vi "refMgr_Example3.vi"() -> ()   [LabVIEW 2017]
uses:
  RefManager/Typedef/RefMgr-Logic-State.ctl
  RefManager/Typedef/RefMgr-StateChangeType.ctl
  RefManager/TagDB RefManager.lvlib
  <userlib>/_NEVSTOP/TagDB/TagDB.lvlib
  UIStateExpression/TagDB UIStateExpression.lvlib
panel:
  in  "aaa":string="aaaa"
  in  "toggle":bool
  in  "stop":bool
  in  "Boolean 0":bool
  in  "StateValue":i32
  in  "Boolean 5":bool
  in  "Boolean 4":bool
  in  "Boolean 3":bool
  in  "Boolean 2":bool
  in  "Boolean 1":bool
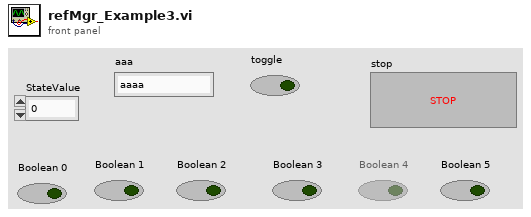
[diagram p1: front panel]
types:
  T1 = typedef "TagDB RefManager.lvlib/RefMgr-Logic-State.ctl" = cluster{"StateName":string, "StateValue":i32, "Type":T2, "Calcs":cluster{"Tag":string, "Exp":string}[]}
  T2 = typedef "TagDB RefManager.lvlib/RefMgr-StateChangeType.ctl" = enum16{"0 - 进入", "1 - 等于", "2 - 退出"}
  T3 = typedef "TagDB.lvlib/TagDB.ctl" = refnum<k1>
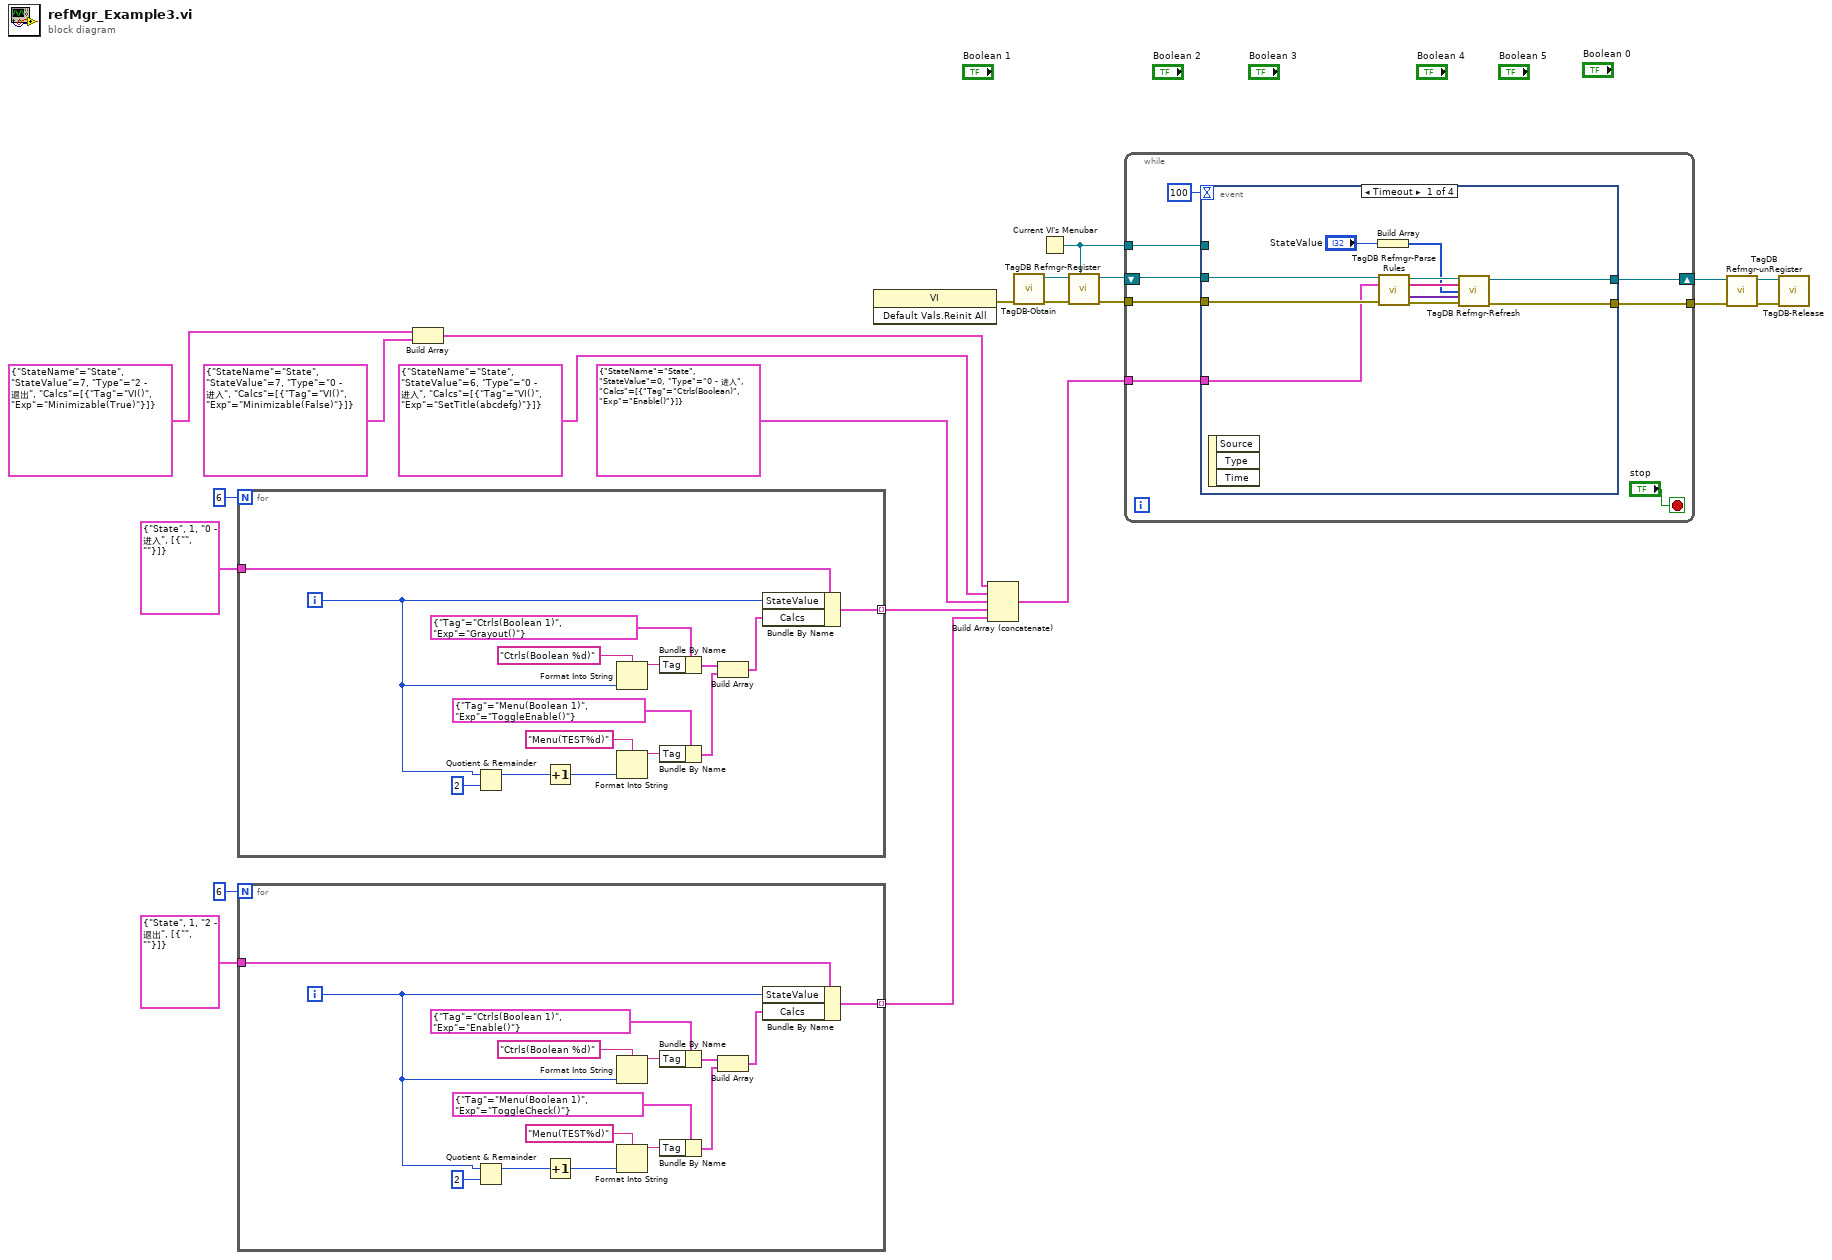
[diagram p0: block diagram]
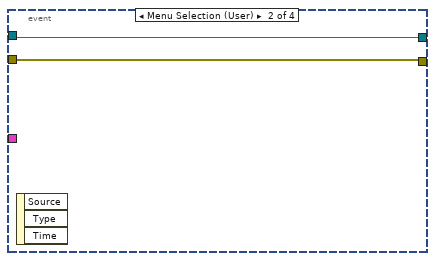
[diagram p2: hidden frame]
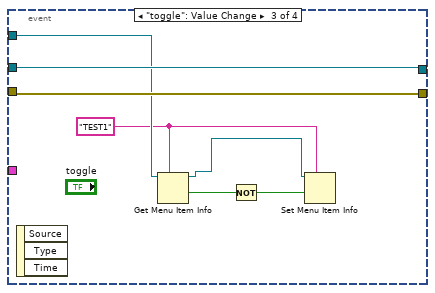
[diagram p3: hidden frame]
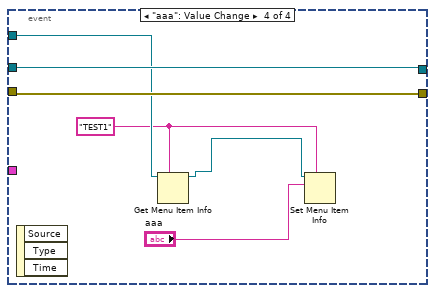
[diagram p4: hidden frame]
diagram:
  n1 = for {
    N: 6 -> [_]
    tunnel: T1 {"StateName"="State", "StateValue"=1, "Type"=enum."0 - 进入", "Calcs"=[{"Tag"="", "Exp"=""}]} ("Cluster") -> [w37]
    tunnel: [w31] -> w16 mode=indexing
    i -> [w27]
    n2 = Quotient & Remainder(x=w27, y=2) -> (x-y*floor(x/y)=w25:i32)  [unwired: 1 out]
    n3 = Increment(x=w25) -> (x+1=w23:i32)
    n4 = Format Into String(format string="Ctrls(Boolean %d)" ("Tag"), w27) -> (resulting string=w34:string)  [unwired: 2 in, 1 out]
    n5 = Format Into String(format string="Menu(TEST%d)" ("Tag"), w23) -> (resulting string=w30:string)  [unwired: 2 in, 1 out]
    n6 = Bundle By Name(cluster=cluster{"Tag":string, "Exp":string} {"Tag"="Ctrls(Boolean 1)", "Exp"="Grayout()"} ("Cluster"), "Tag"=w34) -> (w33:cluster{"Tag":string, "Exp":string})
    n7 = Bundle By Name(cluster=cluster{"Tag":string, "Exp":string} {"Tag"="Menu(Boolean 1)", "Exp"="ToggleEnable()"} ("Cluster"), "Tag"=w30) -> (w24:cluster{"Tag":string, "Exp":string})
    n8 = Build Array(w33, w24) -> (w32:cluster{"Tag":string, "Exp":string}[])
    n9 = Bundle By Name(cluster=w37, "StateValue"=w27, "Calcs"=w32) -> (w31:T1)
  }
  n10 = for {
    N: 6 -> [_]
    tunnel: T1 {"StateName"="State", "StateValue"=1, "Type"=enum."2 - 退出", "Calcs"=[{"Tag"="", "Exp"=""}]} ("Cluster") -> [w52]
    tunnel: [w46] -> w5 mode=indexing
    i -> [w42]
    n11 = Quotient & Remainder(x=w42, y=2) -> (x-y*floor(x/y)=w40:i32)  [unwired: 1 out]
    n12 = Increment(x=w40) -> (x+1=w38:i32)
    n13 = Format Into String(format string="Ctrls(Boolean %d)" ("Tag"), w42) -> (resulting string=w49:string)  [unwired: 2 in, 1 out]
    n14 = Format Into String(format string="Menu(TEST%d)" ("Tag"), w38) -> (resulting string=w45:string)  [unwired: 2 in, 1 out]
    n15 = Bundle By Name(cluster=cluster{"Tag":string, "Exp":string} {"Tag"="Ctrls(Boolean 1)", "Exp"="Enable()"} ("Cluster"), "Tag"=w49) -> (w48:cluster{"Tag":string, "Exp":string})
    n16 = Bundle By Name(cluster=cluster{"Tag":string, "Exp":string} {"Tag"="Menu(Boolean 1)", "Exp"="ToggleCheck()"} ("Cluster"), "Tag"=w45) -> (w39:cluster{"Tag":string, "Exp":string})
    n17 = Build Array(w48, w39) -> (w47:cluster{"Tag":string, "Exp":string}[])
    n18 = Bundle By Name(cluster=w52, "StateValue"=w42, "Calcs"=w47) -> (w46:T1)
  }
  n19 = Build Array(T1 {"StateName"="State", "StateValue"=7, "Type"=enum."2 - 退出", "Calcs"=[{"Tag"="VI()", "Exp"="Minimizable(True)"}]} ("Cluster"), T1 {"StateName"="State", "StateValue"=7, "Type"=enum."0 - 进入", "Calcs"=[{"Tag"="VI()", "Exp"="Minimizable(False)"}]} ("Cluster")) -> (w2:T1[])
  n20 = invoke class="VI" method="Default Vals.Reinit All"() -> (error out=w9:errorcluster)  [unwired: 3 in, 2 out]
  n21 = Build Array (concatenate)(w2, T1 {"StateName"="State", "StateValue"=6, "Type"=enum."0 - 进入", "Calcs"=[{"Tag"="VI()", "Exp"="SetTitle(abcdefg)"}]} ("Cluster"), T1 {"StateName"="State", "StateValue"=0, "Type"=enum."0 - 进入", "Calcs"=[{"Tag"="Ctrls(Boolean)", "Exp"="Enable()"}]} ("Cluster"), w16, w5) -> (w15:T1[])
  n22 = call <userlib>:"TagDB-Obtain.vi"("error in (no error)"=w9) -> ("error out"=w21:errorcluster, "TagDB"=w22:T3)  [unwired: 4 in, 1 out]
  n23 = Current VI's Menubar() -> (w8:refnum<k9>)
  n24 = call "TagDB Refmgr-Register.vi"("menu reference"=w8, "error in (no error)"=w21, "TagDB in"=w22) -> ("error out"=w19:errorcluster, "TagDB out"=w20:T3)  [unwired: 6 in, 1 out]
  n25 = while {
    tunnel: w19 -> [w59]
    tunnel: w15 -> [w58]
    tunnel: [w55] -> w12
    shift-right: [w56] -> w13
    shift-left: w20 -> [w60]
    tunnel: w8 -> [w53]
    stop <- "stop" stop-if-true
    n26 = event shown="[0] Timeout" {
      selector: _ -> [_ _ _ _]
      dyn-events: _ -> [_ _ _ _]
      timeout: 100 -> [_ _ _ _]
      tunnel: w60 -> [w71 w73 w80 w86]
      tunnel: w59 -> [w70 w72 w79 w85]
      tunnel: w58 -> [w69 _ _ _]
      tunnel: [w62 w73 w80 w86] -> w56
      tunnel: [w61 w72 w79 w85] -> w55
      tunnel: w53 -> [_ _ w77 w83]
      event Timeout {
        n27 = event-data() -> ()  [unwired: 1 in, 3 out]
        n28 = Build Array("StateValue") -> (w63:i32[])
        n29 = call "TagDB Refmgr-Parse Rules.vi"("DB Ref"=w71, "Rules"=w69, "error in (no error)"=w70) -> ("DB Ref (dup)"=w68:T3, "StateNames"=w66:string[], "RulesMap"=w65:variant[], "error out"=w67:errorcluster)  [unwired: 9 in]
        n30 = call "TagDB Refmgr-Refresh.vi"("DB Ref"=w68, "StateName"=w66, "State"=w63, "RulesMap"=w65, "error in (no error)"=w67) -> ("DB Ref (dup)"=w62:T3, "error out"=w61:errorcluster)  [unwired: 9 in]
      }
      event Menu Selection (User) {
        n31 = event-data() -> ()  [unwired: 1 in, 3 out]
      }
      event "toggle": Value Change {
        w76 = "TEST1" ("item name")
        n32 = event-data() -> ()  [unwired: 1 in, 3 out]
        n33 = Get Menu Item Info(7:w76, 11:w77) -> (1:w75:bool, 3:w78:refnum<k9>)  [unwired: 1 in, 5 out]
        n34 = Not(x=w75) -> (.not. x?=w74:bool)
        n35 = Set Menu Item Info(7:w76, 9:w74, 11:w78) -> ()  [unwired: 4 in, 2 out]
      }
      event "aaa": Value Change {
        w82 = "TEST1" ("item name")
        n36 = event-data() -> ()  [unwired: 1 in, 3 out]
        n37 = Get Menu Item Info(7:w82, 11:w83) -> (3:w84:refnum<k9>)  [unwired: 1 in, 6 out]
        n38 = Set Menu Item Info(7:w82, 10:"aaa", 11:w84) -> ()  [unwired: 4 in, 2 out]
      }
    }
  }
  n39 = call "TagDB Refmgr-unRegister.vi"("error in (no error)"=w12, "TagDB in"=w13) -> ("error out"=w11:errorcluster, "TagDB out"=w10:T3)  [unwired: 8 in]
  n40 = call <userlib>:"TagDB-Release.vi"("error in (no error)"=w11, "TagDB"=w10) -> ()  [unwired: 9 in, 1 out]
